vi "Configure System Time.vi"(7 "Timezone":string="\"8\", \"1\", \"3.3.0/02\", \"11.2.0/02\"", 8 "error in (no error)":errorcluster, 9 "Real Time":timestamp, 10 "Time Type (0: None)":i32(ring) items=["Real Time", "Timezone"], 11 "VISA resource name":refnum<visa-resource-name>) -> (0 "error out":errorcluster, 3 "VISA resource name out":refnum<visa-resource-name>)   [LabVIEW 2017, in "Keithley 2600 Series.lvlib"]
doc: "Configures the system time."
uses:
  <instrlib>/Keithley 2600 Series/Keithley 2600 Series.lvlib
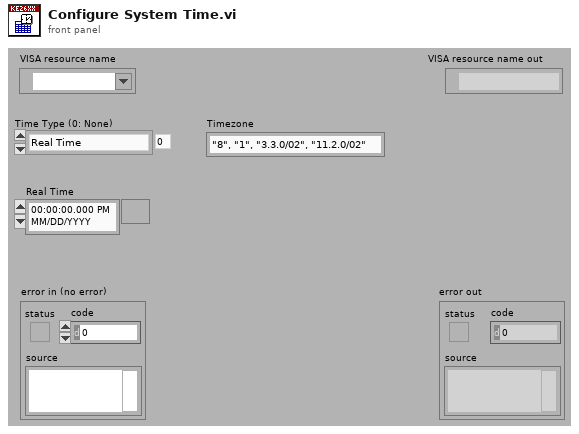
[diagram p1: front panel]
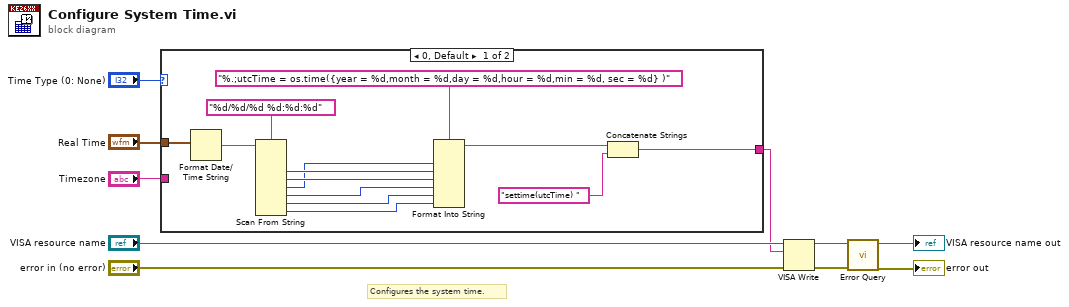
[diagram p0: block diagram]
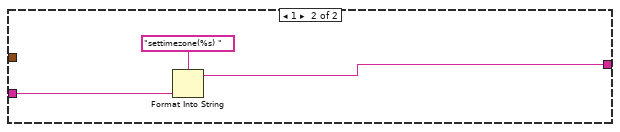
[diagram p2: hidden frame]
diagram:
  # "Configures the system time."
  n1 = case shown="0, Default" "Time Type (0: None)" {
    tunnel: "Real Time" -> [w12 _]
    tunnel: [w11 w24] -> w2
    tunnel: "Timezone" -> [_ w26]
    frame 0, Default {
      n2 = Format Date/Time String(seconds (now)=w12) -> (date/time string=w23:string)  [unwired: 2 in]
      n3 = Scan From String(format string="%d/%d/%d %d:%d:%d", input string=w23) -> (output 1=w20:i32, output 2=w19:i32, output 3=w18:i32, output 4=w17:i32, output 5=w16:i32, output 6=w15:i32)  [unwired: 8 in, 3 out]
      n4 = Format Into String(format string="%.;utcTime = os.time({year = %d,month = %d,day = %d,hour = %d,min = %d, sec = %d} )", w18, w20, w19, w17, w16, w15) -> (resulting string=w14:string)  [unwired: 2 in, 1 out]
      n5 = Concatenate Strings(w14, "settime(utcTime) ") -> (w11:string)
    }
    frame 1 {
      n6 = Format Into String(format string="settimezone(%s) ", w26) -> (resulting string=w24:string)  [unwired: 2 in, 1 out]
    }
  }
  n7 = VISA Write(VISA resource name="VISA resource name", write buffer=w2, error in (no error)="error in (no error)") -> (VISA resource name out=w8:refnum<visa-resource-name>, error out=w7:errorcluster)  [unwired: 1 out]
  n8 = call <instrlib>:"Error Query.vi"("error in (no error)"=w7, "VISA resource name"=w8) -> ("error out"=→"error out":errorcluster, "VISA resource name out"=→"VISA resource name out":refnum<visa-resource-name>)  [unwired: 6 in, 2 out]
